vi "__getDvrData.vi"(8 "error in (no error)":errorcluster, 11 "BME280 in":refnum<class "BME280.lvclass">) -> (0 "error out":errorcluster, 2 "weather":T1, 3 "BME280 out":refnum<class "BME280.lvclass">)   [LabVIEW 2020, in "BME280.lvclass"]
uses:
  BME280.lvclass
  Weather.ctl
  BME280.lvclass/BME280.ctl
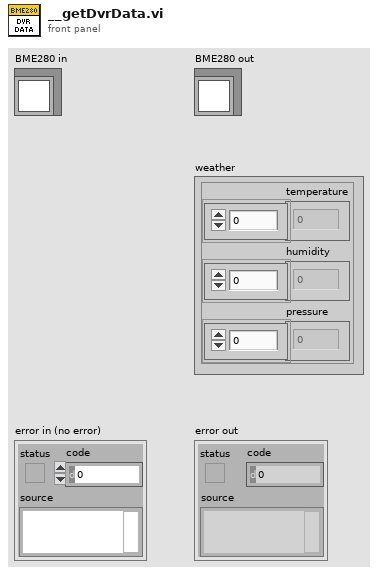
[diagram p1: front panel]
types:
  T1 = typedef "BME280.lvclass/Weather.ctl" = cluster{"temperature":dbl[], "humidity":dbl[], "pressure":dbl[]}
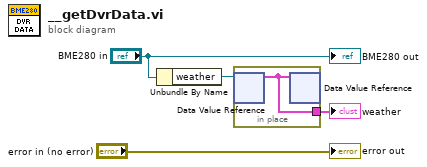
[diagram p0: block diagram]
diagram:
  n1 = Unbundle By Name("BME280 in") -> ("weather"=w4:refnum<data-value>)
  n2 = in-place {
    in-place-border: [w5] -> w3
    n3 = in-place-dvr #1(w4) -> (w5:T1)  [unwired: 1 out]
    n4 = in-place-dvr #1(w5) -> ()  [unwired: 2 out]
  }
  "weather" <- w3
  "error out" <- "error in (no error)"
  "BME280 out" <- "BME280 in"
